vi "Funct Acq Abort actions.vi"() -> (0 "error out":errorcluster)   [LabVIEW 2013]
uses:
  Typedefs/Read Write Enum.ctl
  Typedefs/Top level VI states.ctl
  Global Variables/FPGAstatus_Reference.vi
  <vilib>/rvi/interface/common/niFpgaWaitOnOcc.vi
  <vilib>/Utility/error.llb/Error Cluster From Error Code.vi
  <vilib>/rvi/errors/niLvFpgaAdjustHostInterfaceError.vi
  <vilib>/rvi/interface/nirviReadWriteControl/nirviReadWriteControl.xnode
  RIG-SPECIFIC FILES/FPGA Refs/FPGA Ref.ctl
  NiFpgaLv.dll
  <vilib>/rvi/interface/Simulation/niFpgaSimulationCallBeginRW.vi
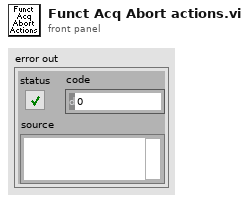
[diagram p1: front panel]
types:
  T1 = typedef "Read Write Enum.ctl" = enum16{"Read", "Write"}
  T2 = typedef "Top level VI states.ctl" = enum16{"None", "Initialise UI", "<STACK PROTOCOL STATES>", "AOL Zstack-START", "AOL Zstack-STOP", "Motor Zstack-START", "Motor Zstack-STOP", "<ACQUISITION PROTOCOL STATES> ", "Functional Acquisition-START", "Functional Acquisition-STOP", "Single Plane Acquisition-START", "Single Plane Acquisition-STOP", "Volume Acquisition-START", "Volume Acquisition-STOP", "<LIVE IMAGING PROTOCOL STATES>", "Live Imaging-START", "Live Imaging-STOP", "Live Plane Imaging-START", "Live Plane Imaging-STOP", "Live Volume Imaging-START", "Live Volume Imaging-STOP", "EXIT"}
  T3 = typedef "FPGA Ref.ctl" = refnum<k20>
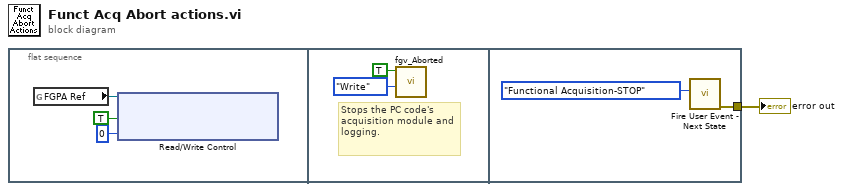
[diagram p0: block diagram]
diagram:
  n1 = flat-sequence {
    tunnel: [w7] -> w1
    frame #0 {
      n2 = global read "FPGAstatus_Reference.vi" "FGPA Ref"() -> (w4:T3)
      n3 = xnode ("Read/Write Control")("FPGA VI Reference In"=w4, "ABORT Trig loop"=TRUE ("ABORT"), "Repeat (Number of Cycles)"=u32 0) -> ()  [unwired: 1 in, 2 out]
    }
    frame #1 {
      # "Stops the PC code's acquisition module and logging."
      n4 = call "fgv_Aborted.vi"("Function"=Read_Write_Enum."Write", "Funct Acq Aborted"=TRUE ("Aborted acquisition")) -> ()  [unwired: 8 in, 2 out]
    }
    frame #2 {
      n5 = call "Fire User Event - Next State.vi"("\"UI Handler loop\" case to execute"=Top_level_VI_states."Functional Acquisition-STOP" ("event data / imaging mode")) -> ("Error Out"=w7:errorcluster)  [unwired: 10 in]
    }
  }
  "error out" <- w1
